vi "Spot Executions.vi"(6 "Reference Value A (0.0)":dbl min=-9.9e+37 max=9.9e+37 step=1.0 format="%.4f", 7 "Reference Value B (0.0)":dbl min=-9.9e+37 max=9.9e+37 step=1.0 format="%.4f", 8 "error in (no error)":errorcluster, 9 "Mode (0: Open)":u32(slide) max=3 step=1, 10 "Spot Number (1)":i16=1 min=1 max=7 step=1, 11 "VISA resource name":refnum<visa-resource-name>) -> (0 "error out":errorcluster, 3 "VISA resource name out":refnum<visa-resource-name>)   [LabVIEW 2016, in "Agilent 428X Series.lvlib"]
doc: "This function executes the OPEN/SHORT/LOAD correction data measurement for the specified frequency point (FREQ1-FREQ7) correction."
uses:
  <instrlib>/Agilent 428X Series/Agilent 428X Series.lvlib
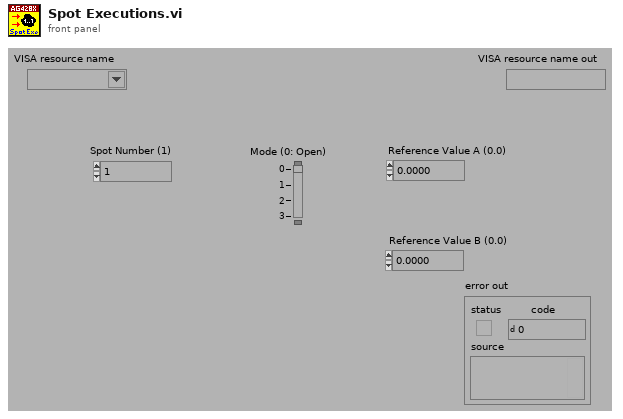
[diagram p1: front panel]
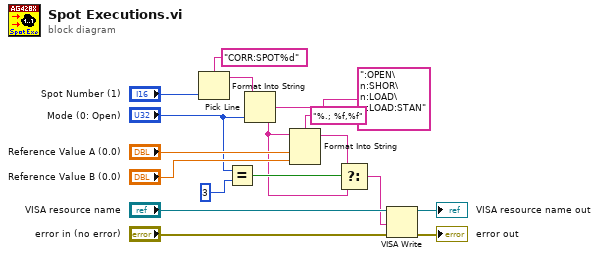
[diagram p0: block diagram]
diagram:
  n1 = Format Into String(format string="CORR:SPOT%d", "Spot Number (1)") -> (resulting string=w15:string)  [unwired: 2 in, 1 out]
  n2 = Equal?(x="Mode (0: Open)", y=u32 3) -> (x = y?=w4:bool)
  n3 = Pick Line(string ("")=w15, multi-line string=":OPEN\n:SHOR\n:LOAD\n:LOAD:STAN", line index="Mode (0: Open)") -> (output string=w2:string)
  n4 = Format Into String(format string="%.; %f,%f", initial string=w2, "Reference Value A (0.0)", "Reference Value B (0.0)") -> (resulting string=w3:string)  [unwired: 1 in, 1 out]
  n5 = Select(t=w3, s=w4, f=w2) -> (s? t:f=w1:string)
  n6 = VISA Write(VISA resource name="VISA resource name", write buffer=w1, error in (no error)="error in (no error)") -> (VISA resource name out=→"VISA resource name out":refnum<visa-resource-name>, error out=→"error out":errorcluster)  [unwired: 1 out]
